vi "Actor Core.vi"(8 "error in":errorcluster, 11 "Example Sink in":refnum<class "Alternative Example Sink.lvclass">) -> (0 "error out":errorcluster, 3 "Actor out":refnum<class "Actor.lvclass">)   [LabVIEW 2016, in "Alternative Example Sink.lvlib" / "Alternative Example Sink.lvclass"]
doc: "(<B>Filename</B>: Actor Framework.lvlib:Actor.lvclass:Actor Core.vi)\n\nReceives messages to the actor, reacts to them, and initiates any error handling that may shut the actor down.\n\nDescendant classes may override this VI to append parallel tasks for the actor to complete while it handles messages. Overrides use the Call Parent Method node."
uses:
  Alternative Example Sink.lvclass
  C:/Program Files (x86)/National Instruments/LabVIEW 2016/vi.lib/ActorFramework/Actor/Actor.lvclass
  C:/Projects/Shared Libraries/Event Actors/Event Sink/Event Sink.lvclass
  <vilib>/ActorFramework/Actor/Actor.lvclass
  Alternative Example Sink.lvclass/Alternative Example Sink.ctl
  <vilib>/ActorFramework/Actor/Actor.lvclass/Actor.ctl
  <vilib>/ActorFramework/Message Enqueuer/Message Enqueuer.lvclass/Message Enqueuer.ctl
  Event Sink/Event Sink.lvclass/Event Sink.ctl
  Event Sink/properties/Read Name.vi
  <vilib>/ActorFramework/Message Enqueuer/Init from Existing Queue.vi
  <vilib>/ActorFramework/Message Enqueuer/Message Enqueuer.lvclass
  Event Sink/Event Sink.lvclass
  Alternative Example Sink Messages/Broadcast Boolean Msg/Broadcast Boolean Msg.lvclass
panel:
  out "Sink Name":string
  in  "Boolean":bool
  out "Time":string
  out "Waveform Graph":dbl[](graph)
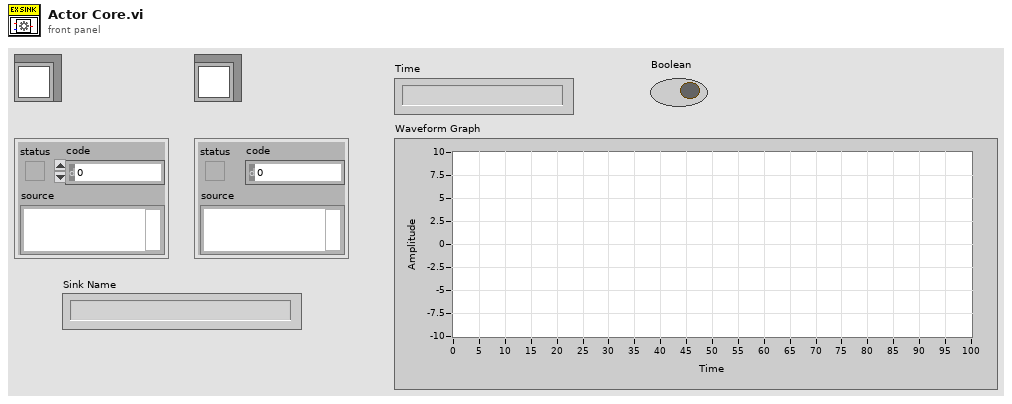
[diagram p1: front panel]
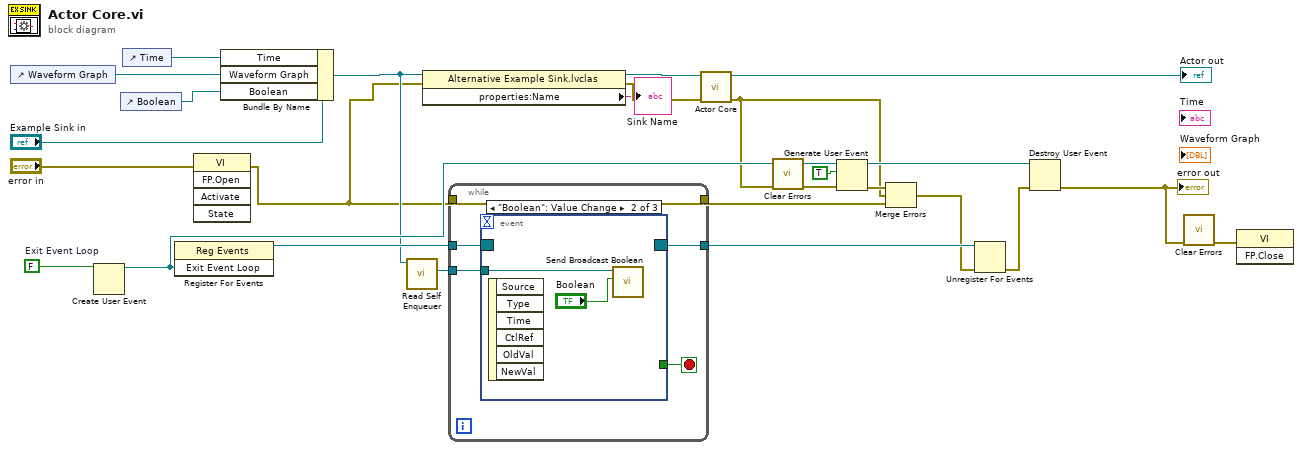
[diagram p0: block diagram]
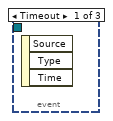
[diagram p2: hidden frame]
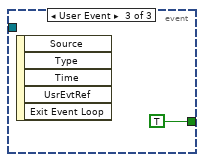
[diagram p3: hidden frame]
diagram:
  w19 = FALSE  # Exit Event Loop
  n1 = control-ref of="Waveform Graph"() -> (w23:refnum<vi>)
  n2 = Create User Event(user event datatype=w19) -> (user event=w16:refnum<user-event>)  [unwired: 1 in, 1 out]
  n3 = control-ref of="Boolean"() -> (w22:refnum<vi>)
  n4 = control-ref of="Time"() -> (w24:refnum<vi>)
  n5 = register-events(w16) -> (reference out=w18:refnum<event-registration>)  [unwired: 2 in, 1 out]
  n6 = invoke class="VI" method="FP.Open"(error in="error in") -> (error out=w3:errorcluster)  [unwired: 4 in, 4 out]
  n7 = Bundle By Name(cluster="Example Sink in", "Time"=w24, "Waveform Graph"=w23, "Boolean"=w22) -> (w11:refnum<class "Alternative Example Sink.lvclass">)
  n8 = call <vilib>:"Read Self Enqueuer.vi"("Actor"=w11) -> ("Self Enqueuer"=w20:refnum<class "Message Enqueuer.lvclass">)  [unwired: 10 in]
  n9 = property class="Alternative Example Sink.lvclas"(reference=w11, error in=w3) -> (reference out=w4:refnum<class "Alternative Example Sink.lvclass">, error out=w2:errorcluster, "properties:Name"=→"Sink Name":string)
  n10 = while {
    tunnel: w20 -> [w31]
    tunnel: w18 -> [w30]
    tunnel: w3 -> [w29]
    tunnel: [w29] -> w10
    tunnel: [w28] -> w14
    stop <- w27 stop-if-true
    n11 = event shown="[1] \"Boolean\": Value Change" {
      selector: w30 -> [_ _ _]
      dyn-events: [_ _ _] -> w28
      timeout: _ -> [_ _ _]
      tunnel: w31 -> [_ w33 _]
      tunnel: [_ _ TRUE] -> w27
      event Timeout {
        n12 = event-data() -> ()  [unwired: 1 in, 3 out]
      }
      event "Boolean": Value Change {
        n13 = event-data() -> ()  [unwired: 1 in, 6 out]
        n14 = call "Send Broadcast Boolean.vi"("Boolean"="Boolean", "Message Enqueuer in"=w33) -> ()  [unwired: 8 in, 2 out]
      }
      event User Event {
        n15 = event-data() -> ()  [unwired: 1 in, 5 out]
      }
    }
  }
  n16 = call-parent "Actor Core.vi"("error in"=w2, "Actor in"=w4) -> ("error out"=w6:errorcluster, "Actor out"=→"Actor out":refnum<class "Actor.lvclass">)  [unwired: 8 in]
  n17 = call <vilib>:"Clear Errors.vi"("error in (no error)"=w6) -> ("error out"=w5:errorcluster)  [unwired: 5 in, 1 out]
  n18 = Generate User Event(user event=w16, event data cluster=TRUE ("event data"), error in=w5) -> (user event out=w15:refnum<user-event>, error out=w17:errorcluster)  [unwired: 1 in]
  n19 = Merge Errors(w17, w6, w10) -> (w7:errorcluster)
  n20 = Unregister For Events(event registration refnum=w14, error in=w7) -> (error out=w13:errorcluster)
  n21 = Destroy User Event(user event=w15, error in=w13) -> (error out=w8:errorcluster)
  "error out" <- w8
  n22 = call <vilib>:"Clear Errors.vi"("error in (no error)"=w8) -> ("error out"=w9:errorcluster)  [unwired: 5 in, 1 out]
  n23 = invoke class="VI" method="FP.Close"(error in=w9) -> ()  [unwired: 2 in, 3 out]
